vi "sub_GSlam_pi2pi.vi"(11 "angle":dbl) -> (3 "result":dbl)   [LabVIEW 2019]
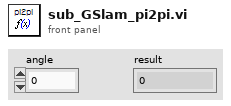
[diagram p1: front panel]
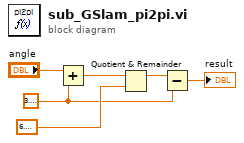
[diagram p0: block diagram]
diagram:
  w2 = 3.141592653589793
  n1 = Add(x="angle", y=w2) -> (x+y=w5:dbl)
  n2 = Quotient & Remainder(x=w5, y=6.283185307179586) -> (x-y*floor(x/y)=w3:dbl)  [unwired: 1 out]
  n3 = Subtract(x=w3, y=w2) -> (x-y=→"result":dbl)
